vi "Get MFC Instance.vi"(8 "error in":errorcluster, 11 "CRDS in":refnum<class "CRDS.lvclass">) -> (0 "error out":errorcluster, 2 "MFCs":refnum<class "Serial IO.lvclass">, 3 "CRDS out":refnum<class "CRDS.lvclass">)   [LabVIEW 2011, in "CRDS.lvclass"]
uses:
  CRDS.lvclass
  Reusable/Serial IO/Base/Serial IO.lvclass
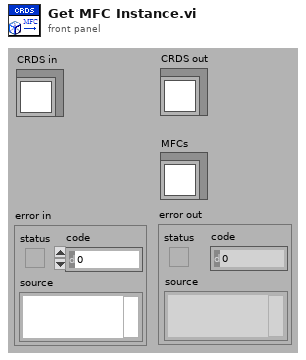
[diagram p1: front panel]
types:
  T1 = cluster{"YAG Ctr":refnum<k21>, "Diode Ctr":refnum<k21>, "Gated Ctr":refnum<k21>, "LF AI":refnum<k21>, "HF AI":refnum<k21>, "valveIn":refnum<k21>, "valveOut":refnum<k21>}
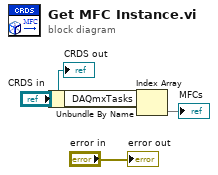
[diagram p0: block diagram]
diagram:
  n1 = Unbundle By Name("CRDS in") -> ("DAQmxTasks"=w1:T1)
  n2 = Index Array(array=w1) -> (element=→"MFCs")  [unwired: 1 in]
  "error out" <- "error in"
  "CRDS out" <- "CRDS in"
